vi "2017-01-18 Scan.vi"() -> ()   [LabVIEW 2016]
uses:
  <vilib>/Utility/error.llb/DialogType.ctl
  <vilib>/DAQmx/write.llb/DAQmx Write (Analog DBL 1Chan 1Samp).vi
  <vilib>/DAQmx/create/channels.llb/DAQmx Create Channel (AO-Voltage-Basic).vi
  <vilib>/DAQmx/miscellaneous.llb/DAQmx Fill In Error Info.vi
panel:
  out "Next Voltage":dbl
  out "Current Voltage":dbl
  in  "Voltage Step":dbl=0.1
  in  "Physical Channel(s)":tag="Dev1/ao0"
  in  "Min Voltage Voltage":dbl=-10.0
  in  "Max Voltage":dbl=10.0
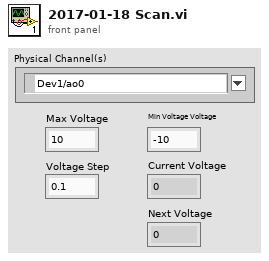
[diagram p1: front panel]
types:
  T1 = typedef "DialogType.ctl" = u16
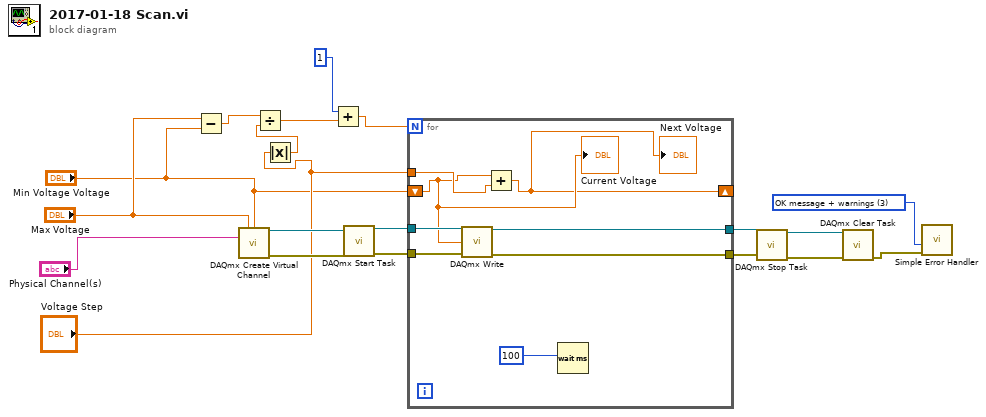
[diagram p0: block diagram]
diagram:
  w10 = T1 3 items=["no dialog", "OK message", "continue or stop message", "OK message + warnings", "continue/stop + warnings"] ("type of dialog (OK msg:1)")
  n1 = Subtract(x="Max Voltage", y="Min Voltage Voltage") -> (x-y=w7:dbl)
  n2 = call-poly <vilib>:"DAQmx Create Virtual Channel.vi"("maximum value"="Max Voltage", "minimum value"="Min Voltage Voltage", "physical channels"="Physical Channel(s)") -> ("task out"=w18:refnum<k21>, "error out"=w17:errorcluster)  [unwired: 11 in]
  n3 = Absolute Value(x="Voltage Step") -> (abs(x)=w5:dbl)
  n4 = Divide(x=w7, y=w5) -> (x/y=w3:dbl)
  n5 = Add(x=1, y=w3) -> (x+y=w1:dbl)
  n6 = call <vilib>:"DAQmx Start Task.vi"("task/channels in"=w18, "error in"=w17) -> ("task out"=w16:refnum<k21>, "error out"=w15:errorcluster)  [unwired: 12 in]
  n7 = for {
    N: w1 -> [_]
    tunnel: w16 -> [w27]
    tunnel: w15 -> [w26]
    tunnel: [w25] -> w14
    tunnel: [w22] -> w13
    tunnel: "Voltage Step" -> [w24]
    shift-right: [w20] -> _
    shift-left: "Min Voltage Voltage" -> [w21]
    n8 = call-poly <vilib>:"DAQmx Write.vi"("task/channels in"=w27, "data"=w21, "error in"=w26) -> ("task out"=w22:refnum<k21>, "error out"=w25:errorcluster)  [unwired: 10 in, 1 out]
    n9 = Add(x=w21, y=w24) -> (x+y=w20:dbl)
    "Next Voltage" <- w20
    n10 = Wait (ms)(milliseconds to wait=100) -> ()  [unwired: 1 out]
    "Current Voltage" <- w21
  }
  n11 = call <vilib>:"DAQmx Stop Task.vi"("task/channels in"=w13, "error in"=w14) -> ("task out"=w11:refnum<k21>, "error out"=w12:errorcluster)  [unwired: 12 in]
  n12 = call <vilib>:"DAQmx Clear Task.vi"("task in"=w11, "error in"=w12) -> ("error out"=w9:errorcluster)  [unwired: 13 in]
  n13 = call <vilib>:"Simple Error Handler.vi"("type of dialog (OK msg:1)"=w10, "error in (no error)"=w9) -> ()  [unwired: 3 in, 5 out]
